vi "New User Event.vi"(8 "error in (no error)":errorcluster) -> (0 "error out":errorcluster, 3 "user event":refnum<user-event>)   [LabVIEW 2021, in "Architecture.lvlib" / "Message.lvclass"]
doc: "Creates a message user event."
uses:
  Message.lvclass
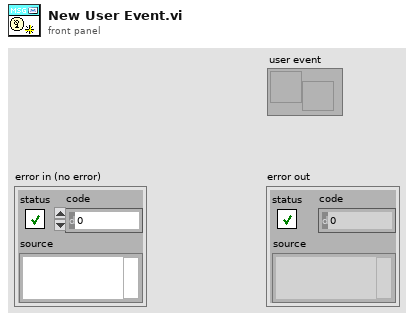
[diagram p1: front panel]
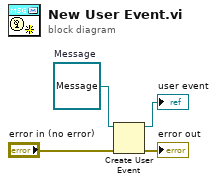
[diagram p0: block diagram]
diagram:
  w2 = refnum<class "Message.lvclass"> refnum  # Message
  n1 = Create User Event(user event datatype=w2, error in="error in (no error)") -> (user event=→"user event":refnum<user-event>, error out=→"error out":errorcluster)
